vi "Get Path to Plugins Folder.vi"(8 "error in (no error)":errorcluster, 11 "Data Sharing Framework in":refnum<class "Framework.lvclass">) -> (0 "error out":errorcluster, 1 "found?":bool, 2 "plugins folder path":path, 3 "Data Sharing Framework out":refnum<class "Framework.lvclass">, 5 "version year":string)   [LabVIEW 2016, in "Framework.lvclass"]
uses:
  Framework.lvclass
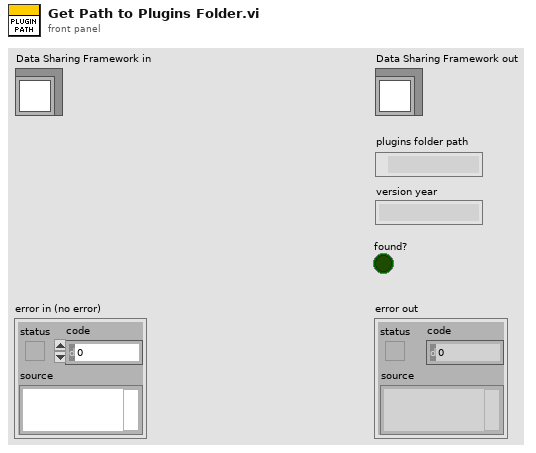
[diagram p1: front panel]
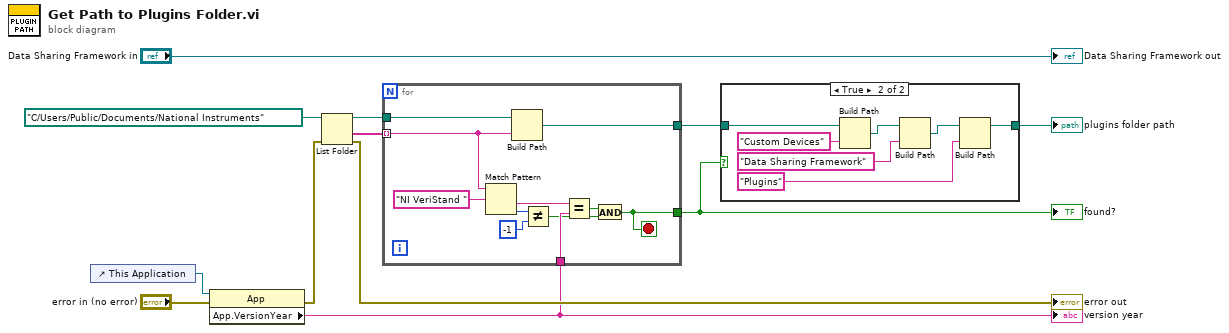
[diagram p0: block diagram]
diagram:
  n1 = control-ref of="This Application"() -> (w8:refnum<vi>)
  n2 = property class="App"(reference=w8, error in="error in (no error)") -> (error out=w7:errorcluster, "App.VersionYear"=w4:string)  [unwired: 1 out]
  "version year" <- w4
  n3 = List Folder(path=path "C:/Users/Public/Documents/National Instruments", error in=w7) -> (path out=w9:path, folder names=w10:string[], error out=→"error out":errorcluster)  [unwired: 2 in, 1 out]
  n4 = for {
    tunnel: w10 -> [w19] mode=indexing
    tunnel: w9 -> [w20]
    tunnel: w4 -> [w16]
    tunnel: [w14] -> w3
    tunnel: [w13] -> w2
    stop <- w13 stop-if-true
    n5 = Match Pattern(string=w19, regular expression="NI VeriStand ") -> (after substring=w18:string, offset past match=w22:i32)  [unwired: 1 in, 2 out]
    n6 = Build Path(base path=w20, name or relative path=w19) -> (appended path=w14:path)
    n7 = Not Equal?(x=w22, y=-1) -> (x != y?=w15:bool)
    n8 = Equal?(x=w18, y=w16) -> (x = y?=w17:bool)
    n9 = And(x=w17, y=w15) -> (x .and. y?=w13:bool)
  }
  "found?" <- w2
  n10 = case shown="True" w2 {
    tunnel: w3 -> [w24 w31]
    tunnel: [w24 w25] -> w1
    frame False {
    }
    frame True {
      n11 = Build Path(base path=w31, name or relative path="Custom Devices") -> (appended path=w29:path)
      n12 = Build Path(base path=w29, name or relative path="Data Sharing Framework") -> (appended path=w27:path)
      n13 = Build Path(base path=w27, name or relative path="Plugins") -> (appended path=w25:path)
    }
  }
  "plugins folder path" <- w1
  "Data Sharing Framework out" <- "Data Sharing Framework in"
